vi "Sequence.BuildPreviewiStep.vi"(8 "Step":T1, 9 "Step IO":cluster{"Ramp Pattern":dbl[]}, 10 "iStep Iterations":i32, 11 "Step Duration":u64) -> (3 "Ramp Pattern":dbl[](array[numeric]))   [LabVIEW 2013, in "Simple Sequence Tools - Shared.lvlib"]
uses:
  Simple Sequence Tools - Shared.lvlib
  Types/Step.Types.ctl
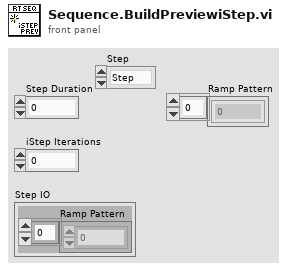
[diagram p1: front panel]
types:
  T1 = typedef "Simple Sequence Tools - Shared.lvlib/Step.Types.ctl" = enum8{"Step", "iStep", "Ramp", "Unchanged", "Unknown", "Sine", "LogSine", "LinearSine", "ForcedRamp"}
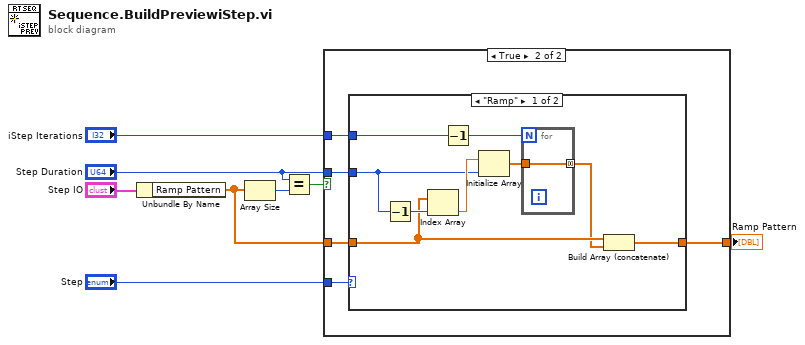
[diagram p0: block diagram]
diagram:
  n1 = Unbundle By Name("Step IO") -> ("Ramp Pattern"=w6:dbl[])
  n2 = Array Size(array=w6) -> (size(s)=w2:i32)
  n3 = Equal?(x="Step Duration", y=w2) -> (x = y?=w7:bool)
  n4 = case shown="True" w7 {
    tunnel: "iStep Iterations" -> [_ w14]
    tunnel: w6 -> [w9 w13]
    tunnel: [w9 w12] -> w8
    tunnel: "Step" -> [_ w11]
    tunnel: "Step Duration" -> [_ w10]
    frame False {
    }
    frame True {
      n5 = case shown="\"Ramp\"" w11 {
        tunnel: w14 -> [w23 w27]
        tunnel: w13 -> [w18 w26]
        tunnel: [w16 w25] -> w12
        tunnel: w10 -> [w15 _]
        frame "Ramp" {
          n6 = Decrement(x=w15) -> (x-1=w21:u64)
          n7 = Index Array(array=w18, index=w21) -> (element=w20:dbl)
          n8 = Decrement(x=w23) -> (x-1=w22:i32)
          n9 = Initialize Array(w20, w15) -> (w19:dbl[])
          n10 = for {
            N: w22 -> [_]
            tunnel: w19 -> [w24]
            tunnel: [w24] -> w17 mode=concatenating
          }
          n11 = Build Array (concatenate)(w18, w17) -> (w16:dbl[])
        }
        frame Default {
          n12 = for {
            N: w27 -> [_]
            tunnel: w26 -> [w28]
            tunnel: [w28] -> w25 mode=concatenating
          }
        }
      }
    }
  }
  "Ramp Pattern" <- w8
